vi "main.vi"() -> ()   [LabVIEW 2013]
uses:
  Global 1.vi
panel:
  out "?":picture
  out "?":picture
  out "Current Time":timestamp format="%<%I:%M:%S %p\n%x>T"
  in  "Initialize":bool
  in  "Clean":bool
  in  "stop":bool
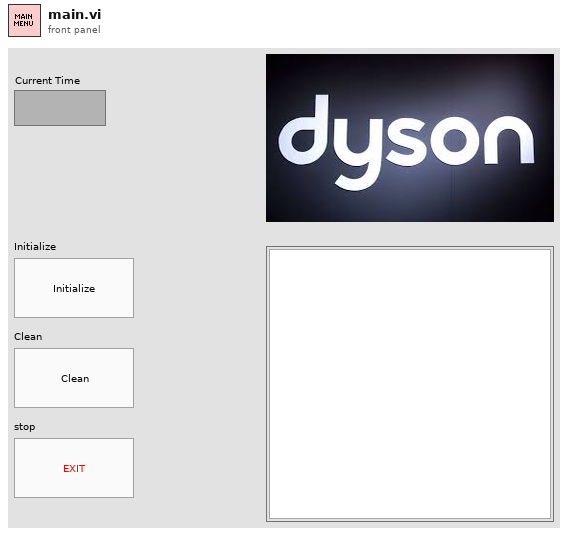
[diagram p1: front panel]
types:
  T1 = enum8{"Enabled", "Disabled", "Disabled and Grayed Out"}
  T2 = typedef "imagedata.ctl" = cluster{"image type":i32, "image depth":i32, "image":u8[], "mask":u8[], "colors":u32[], "Rectangle":cluster{"left":i16, "top":i16, "right":i16, "bottom":i16}}
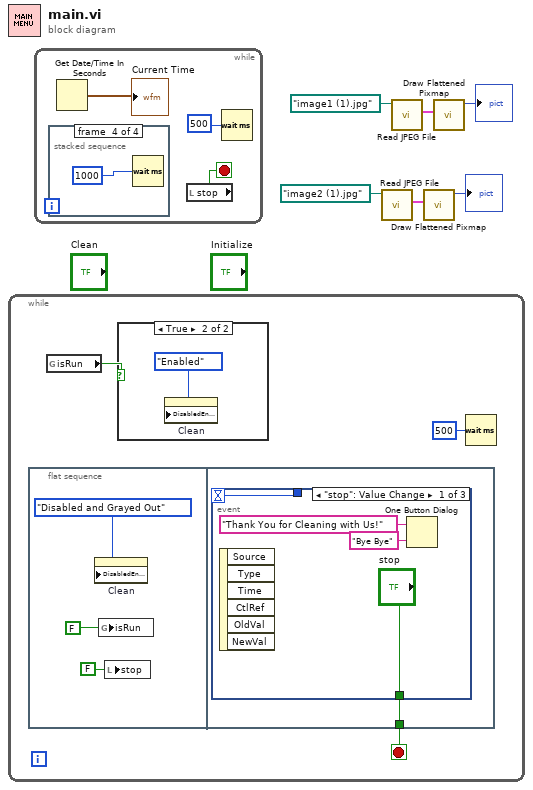
[diagram p0: block diagram]
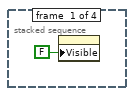
[diagram p2: hidden frame]
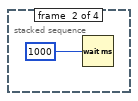
[diagram p3: hidden frame]
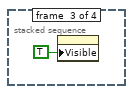
[diagram p4: hidden frame]
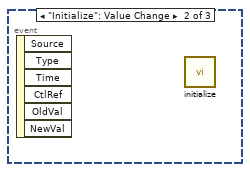
[diagram p6: hidden frame]
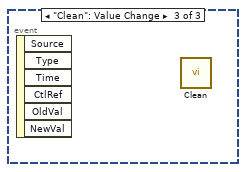
[diagram p7: hidden frame]
diagram:
  n1 = while {
    stop <- w7 stop-if-true
    n2 = flat-sequence {
      tunnel: [w14] -> w7
      frame #0 {
        n3 = property on="Clean" class="Bool"("DisabledEnum"=T1."Disabled and Grayed Out" ("Disabled")) -> ()  [unwired: 2 in, 2 out]
        n4 = global write "Global 1.vi" "isRun"(FALSE ("IsRun")) -> ()
        n5 = local write "stop"(FALSE ("stop")) -> ()
      }
      frame #1 {
        n6 = event shown="[0] \"stop\": Value Change" {
          selector: _ -> [_ _ _]
          dyn-events: _ -> [_ _ _]
          timeout: _ -> [w18 _ _]
          tunnel: [w18 _ _] -> _
          tunnel: ["stop" _ _] -> w14
          event "stop": Value Change {
            n7 = event-data() -> ()  [unwired: 1 in, 6 out]
            n8 = One Button Dialog(message="Thank You for Cleaning with Us!", button name ("OK")="Bye Bye") -> ()  [unwired: 1 out]
          }
          event "Initialize": Value Change {
            n9 = event-data() -> ()  [unwired: 1 in, 6 out]
            n10 = call "initialize.vi"() -> ()  [unwired: 1 in]
          }
          event "Clean": Value Change {
            n11 = event-data() -> ()  [unwired: 1 in, 6 out]
            n12 = call "Clean.vi"() -> ()  [unwired: 1 in]
          }
        }
      }
    }
    n13 = global read "Global 1.vi" "isRun"() -> (w8:bool)
    n14 = case shown="True" w8 {
      frame False {
      }
      frame True {
        n15 = property on="Clean" class="Bool"("DisabledEnum"=T1."Enabled" ("Disabled")) -> ()  [unwired: 2 in, 2 out]
      }
    }
    n16 = Wait (ms)(milliseconds to wait=u32 500) -> ()  [unwired: 1 out]
  }
  n17 = while {
    stop <- w20 stop-if-true
    n18 = stacked-sequence {
      frame #0 {
        n19 = property class="Pict"("Visible"=FALSE) -> ()  [unwired: 2 in, 2 out]
      }
      frame #1 {
        n20 = Wait (ms)(milliseconds to wait=u32 1000 ("millisecond timer value")) -> ()  [unwired: 1 out]
      }
      frame #2 {
        n21 = property class="Pict"("Visible"=TRUE) -> ()  [unwired: 2 in, 2 out]
      }
      frame #3 {
        n22 = Wait (ms)(milliseconds to wait=u32 1000 ("millisecond timer value")) -> ()  [unwired: 1 out]
      }
    }
    n23 = Get Date/Time In Seconds() -> (seconds since 1Jan1904=→"Current Time":timestamp)
    n24 = local read "stop"() -> (w20:bool)
    n25 = Wait (ms)(milliseconds to wait=u32 500 ("millisecond timer value")) -> ()  [unwired: 1 out]
  }
  n26 = call <vilib>:"Read JPEG File.vi"("path to JPEG file"=path "image2 (1).jpg") -> ("image data"=w5:T2)  [unwired: 8 in, 2 out]
  n27 = call <vilib>:"Read JPEG File.vi"("path to JPEG file"=path "image1 (1).jpg") -> ("image data"=w2:T2)  [unwired: 8 in, 2 out]
  n28 = call <vilib>:"Draw Flattened Pixmap.vi"("image data"=w5) -> ("new picture"=→"?":picture)  [unwired: 8 in]
  n29 = call <vilib>:"Draw Flattened Pixmap.vi"("image data"=w2) -> ("new picture"=→"?":picture)  [unwired: 8 in]
